vi "StateAlarmManagement.vi"(0 "Master State In":T1(ring)) -> ()   [LabVIEW 2020]
doc: "This VI manages the Master ALARM and master CAUTION states for the robot."
uses:
  GlobalPoseAndTargeting.vi
  GlobalDriverStationData.vi
  GlobalAutonomous.vi
  GlobalDrivebase.vi
  GlobalMiscellaneous.vi
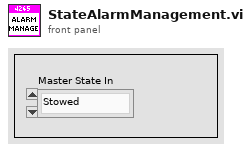
[diagram p1: front panel]
types:
  T1 = enum16{"Stowed", "Balancing", "Scoring", "Hoppering", "Ground", "Shelf"}
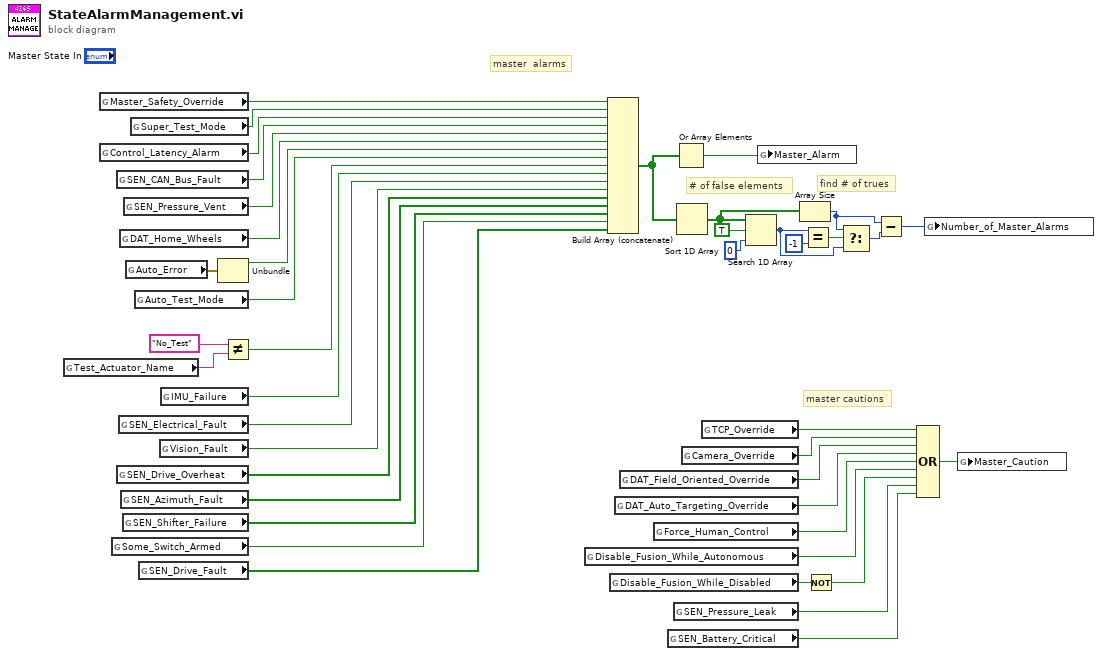
[diagram p0: block diagram]
diagram:
  # "master cautions"
  # "master  alarms"
  # "# of false elements"
  # "find # of trues"
  n1 = global read "GlobalDriverStationData.vi" "Test_Actuator_Name"() -> (w36:string)
  n2 = global read "GlobalDriverStationData.vi" "Master_Safety_Override"() -> (w42:bool)
  n3 = global read "GlobalMiscellaneous.vi" "Control_Latency_Alarm"() -> (w17:bool)
  n4 = global read "GlobalDriverStationData.vi" "Some_Switch_Armed"() -> (w11:bool)
  n5 = global read "GlobalMiscellaneous.vi" "SEN_CAN_Bus_Fault"() -> (w16:bool)
  n6 = global read "GlobalDrivebase.vi" "SEN_Drive_Overheat"() -> (w14:bool[])
  n7 = global read "GlobalMiscellaneous.vi" "SEN_Electrical_Fault"() -> (w18:bool)
  n8 = global read "GlobalDrivebase.vi" "DAT_Home_Wheels"() -> (w19:bool)
  n9 = global read "GlobalDrivebase.vi" "SEN_Azimuth_Fault"() -> (w13:bool[])
  n10 = global read "GlobalDrivebase.vi" "SEN_Shifter_Failure"() -> (w12:bool[])
  n11 = global read "GlobalMiscellaneous.vi" "SEN_Pressure_Vent"() -> (w15:bool)
  n12 = global read "GlobalAutonomous.vi" "Auto_Error"() -> (w40:errorcluster)
  n13 = global read "GlobalDriverStationData.vi" "Super_Test_Mode"() -> (w41:bool)
  n14 = global read "GlobalDriverStationData.vi" "Auto_Test_Mode"() -> (w38:bool)
  n15 = global read "GlobalDrivebase.vi" "SEN_Drive_Fault"() -> (w1:bool[])
  n16 = global read "GlobalPoseAndTargeting.vi" "Vision_Fault"() -> (w33:bool)
  n17 = global read "GlobalPoseAndTargeting.vi" "IMU_Failure"() -> (w34:bool)
  n18 = Unbundle(w40) -> ("status"=w39:bool)  [unwired: 2 out]
  n19 = Not Equal?(x="No_Test", y=w36) -> (x != y?=w35:bool)
  n20 = global read "GlobalDriverStationData.vi" "Disable_Fusion_While_Autonomous"() -> (w6:bool)
  n21 = Build Array (concatenate)(w42, w41, w17, w16, w15, w19, w39, w38, w35, w34, w18, w33, w14, w13, w12, w11, w1) -> (w24:bool[])
  n22 = global read "GlobalDriverStationData.vi" "Disable_Fusion_While_Disabled"() -> (w5:bool)
  n23 = global read "GlobalDrivebase.vi" "DAT_Auto_Targeting_Override"() -> (w8:bool)
  n24 = global read "GlobalDrivebase.vi" "DAT_Field_Oriented_Override"() -> (w9:bool)
  n25 = global read "GlobalDriverStationData.vi" "Force_Human_Control"() -> (w7:bool)
  n26 = global read "GlobalMiscellaneous.vi" "SEN_Battery_Critical"() -> (w2:bool)
  n27 = global read "GlobalMiscellaneous.vi" "SEN_Pressure_Leak"() -> (w3:bool)
  n28 = Or Array Elements(Boolean array=w24) -> (logical OR=w23:bool)
  n29 = Sort 1D Array(array=w24) -> (sorted array=w29:bool[])
  n30 = global read "GlobalDriverStationData.vi" "Camera_Override"() -> (w10:bool)
  n31 = global read "GlobalDriverStationData.vi" "TCP_Override"() -> (w21:bool)
  n32 = Search 1D Array(1D array=w29, element=TRUE, start index (0)=0) -> (index of element=w32:i32)
  n33 = global write "GlobalMiscellaneous.vi" "Master_Alarm"(w23) -> ()
  n34 = Array Size(array=w29) -> (size(s)=w31:i32)
  n35 = Equal?(x=w32, y=-1) -> (x = y?=w28:bool)
  n36 = Not(x=w5) -> (.not. x?=w4:bool)
  n37 = Select(t=w31, s=w28, f=w32) -> (s? t:f=w30:i32)
  n38 = Subtract(x=w31, y=w30) -> (x-y=w22:i32)
  n39 = Compound Arithmetic op=OR(w21, w10, w9, w8, w7, w6, w4, w3, w2) -> (w20:bool)
  n40 = global write "GlobalMiscellaneous.vi" "Number_of_Master_Alarms"(w22) -> ()
  n41 = global write "GlobalMiscellaneous.vi" "Master_Caution"(w20) -> ()
